vi "Case_Structure_Motor_Control 1.vi"   [LabVIEW 2012]
doc: "This example is for the LEGO MINDSTORMS NXT. The program demonstrates how a case structure can be used to control the movement of a motor. The state of the case structure is determined by the feedback from a touch sensor."
uses:
  <vilib>/NXT/Block Support/NXT_InputPort.ctl
  <vilib>/NXT/Dual Mode Library/Motors/MotorOn.vi
  <vilib>/NXT/Dual Mode Library/BT/BlueTooth_Write_String_toComputer.vi
  <vilib>/NXT/Dual Mode Library/Motors/MotorBrake.vi
panel:
  # "Case Structure Control"
  # "DESCRIPTION\n\nThis example demonstrates how a case structure can be used to control the movement of a motor. The state of the case structure is determined by the feedback from a touch sensor.\n\nPORTS \n\nPort A: motor\nPort 1: touch sensor\n\nTIPS \n\n- CTRL-E to open the block diagram. \n- This program can be executed in direct or remote mode."
types:
  T1 = typedef "NXT_InputPort.ctl" = u8
  T2 = typedef "LVHSConnector.ctl" = refnum<class "BrickReference.lvclass">
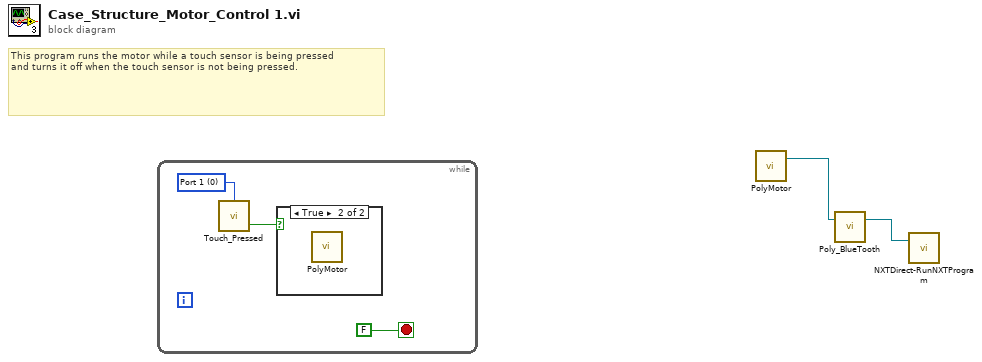
[diagram p0: block diagram]
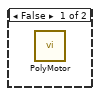
[diagram p2: hidden frame]
diagram:
  # "This program runs the motor while a touch sensor is being pressed \nand turns it off when the touch sensor is not being pressed."
  n1 = while {
    stop <- FALSE stop-if-true
    w4 = T1 0 items=["Port 1", "Port 2", "Port 3", "Port 4"] ("Port (Port 1)")
    n2 = call <vilib>:"Touch_Pressed.vi"("Port (Port 1)"=w4) -> ("Yes / No"=w5:bool)  [unwired: 2 in, 1 out]
    n3 = case shown="True" w5 {
      frame False {
        n4 = call-poly <vilib>:"PolyMotor.vi"() -> ()  [unwired: 4 in, 1 out]
      }
      frame True {
        n5 = call-poly <vilib>:"PolyMotor.vi"() -> ()  [unwired: 4 in, 1 out]
      }
    }
  }
  n6 = call-poly <vilib>:"PolyMotor.vi"() -> ("NXT"=w2:T2)  [unwired: 4 in]
  n7 = call-poly <vilib>:"Poly_BlueTooth.vi"("NXT"=w2) -> ("NXT"=w1:T2)  [unwired: 3 in]
  n8 = call <vilib>:"NXTDirect-RunNXTProgram.vi"("NXT"=w1) -> ()  [unwired: 3 in, 1 out]
